vi "CLIENT_show_hide_pages.vi"(7 "This VI":refnum<vi>, 10 "visible_pages":T1(array[ring]), 11 "main_tab_ref":refnum<vi>) -> ()   [LabVIEW 2020]
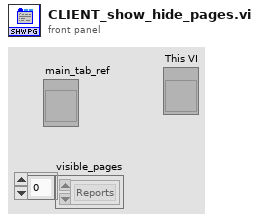
[diagram p1: front panel]
types:
  T1 = enum32{"Reports", "Reference Editor", "Archivisation Editor", "User Management", "Manual SQL Requests", "Text SQL Requests", "Errors"}[]
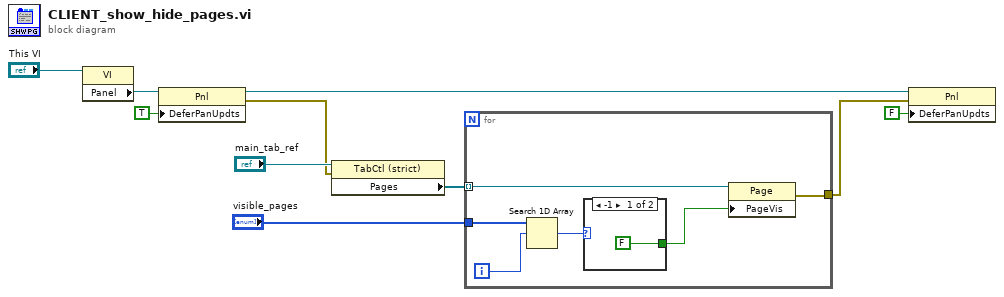
[diagram p0: block diagram]
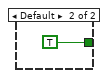
[diagram p2: hidden frame]
diagram:
  n1 = property class="VI"(reference="This VI") -> ("Panel"=w6:refnum<vi>)  [unwired: 1 in, 2 out]
  n2 = property class="Pnl"(reference=w6, "DeferPanUpdts"=TRUE ("Defer Panel Updates")) -> (reference out=w2:refnum<vi>, error out=w4:errorcluster)  [unwired: 1 in]
  n3 = property class="TabCtl (strict)"(reference="main_tab_ref", error in=w4) -> ("Pages"=w10:refnum<vi>[])  [unwired: 2 out]
  n4 = for {
    tunnel: w10 -> [w15] mode=indexing
    tunnel: "visible_pages" -> [w14]
    tunnel: [w11] -> w1
    i -> [w13]
    n5 = Search 1D Array(1D array=w14, element=w13) -> (index of element=w12:i32)  [unwired: 1 in]
    n6 = case shown="-1" w12 {
      tunnel: [FALSE ("Page Visible") TRUE ("Page Visible")] -> w16
      frame -1 {
      }
      frame Default {
      }
    }
    n7 = property class="Page"(reference=w15, "PageVis"=w16) -> (error out=w11:errorcluster)  [unwired: 1 in, 1 out]
  }
  n8 = property class="Pnl"(reference=w2, error in=w1, "DeferPanUpdts"=FALSE ("Defer Panel Updates")) -> ()  [unwired: 2 out]
